vi "Teleop.vi"(10 "Match Info":T5={"Autonomous Elapsed Seconds"=0.0, "TeleOp Elapsed Seconds"=0.0, "Disabled Elapsed Seconds"=0.0, "Visited Autonomous"=FALSE, "Visited TeleOp"=FALSE, "Visited Disabled"=FALSE, "Autonomous Settings"={"Autonomous Style"=enum."Independent", "VI Refnum"=refnum}}, 11 "Call Context":T6) -> ()   [LabVIEW 2013]
doc: "This VI is called for each TeleOp packet received from the DS where the robot is not disabled. It is often used to read from the joysticks and update I/O or to update setpoints for timed control loops. It should complete and return within 20 milliseconds or it may miss DS packets."
uses:
  <vilib>/Rock Robotics/WPI/DriverStation/WPI_DriverStationDerivedRobotMode.ctl
  <vilib>/Rock Robotics/WPI/DriverStation/WPI_DriverStationMatch Info.ctl
  <vilib>/Rock Robotics/WPI/Joystick/WPI_JoystickButtonState.ctl
  <vilib>/Rock Robotics/WPI/Solenoid/WPI_SolenoidValue.ctl
  <vilib>/Rock Robotics/WPI/Relay/WPI_RelayValue.ctl
  Robot Global Data.vi
  <vilib>/Rock Robotics/Network Tables/SD Read Number.vi
  <vilib>/Rock Robotics/WPI/Solenoid/WPI_SolenoidGetEnum.vi
  <vilib>/Rock Robotics/WPI/Solenoid/Deprecated/WPI_SolenoidGetBool.vi
  <vilib>/Rock Robotics/WPI/Compressor/WPI_CompressorGetSetRefNum.vi
  <vilib>/Rock Robotics/WPI/Solenoid/WPI_SolenoidSetEnum.vi
  <vilib>/Rock Robotics/WPI/Joystick/WPI_JoystickGetSetRefNum.vi
  <vilib>/Rock Robotics/WPI/RobotDrive/WPI_RobotDriveGetSetRefNum.vi
panel:
  out "Waveform Chart 3":dbl(graph)
  out "Buttons":T1
  out "Axes":T2
  out "Firing Pin on off":bool
  out "Reed Switch 2":bool
  out "Reed Switch 1":bool
  out "Top Limit Tripped":bool
  out "Micro Switch":bool
  out "Bottom Limit Tripped":bool
  in  "Grabber Axis Value":T3(ring)
  out "Waveform Chart 2":dbl(graph)
  in  "OK Button":bool
  in  "Set Point":dbl
  in  "Run Grabber PID":bool
  in  "Current Shooter Status":T4(ring)
  out "Waveform Chart":dbl(graph)
  out "Mechanism Moving Up":bool
  out "Mechanism Moving Down":bool
  out "Time Since Button Pressed":dbl
  in  "Manual Override Activated":bool
  in  "Button 8 Pressed":bool
  in  "Button 3 Pressed":bool
  in  "Button 2 Pressed":bool
  in  "Tick Taken":bool
  out "Time at Gather":dbl
  out "Timer for firing mech":dbl
  in  "Mechanism Status":string
  # "Joystick Debug"
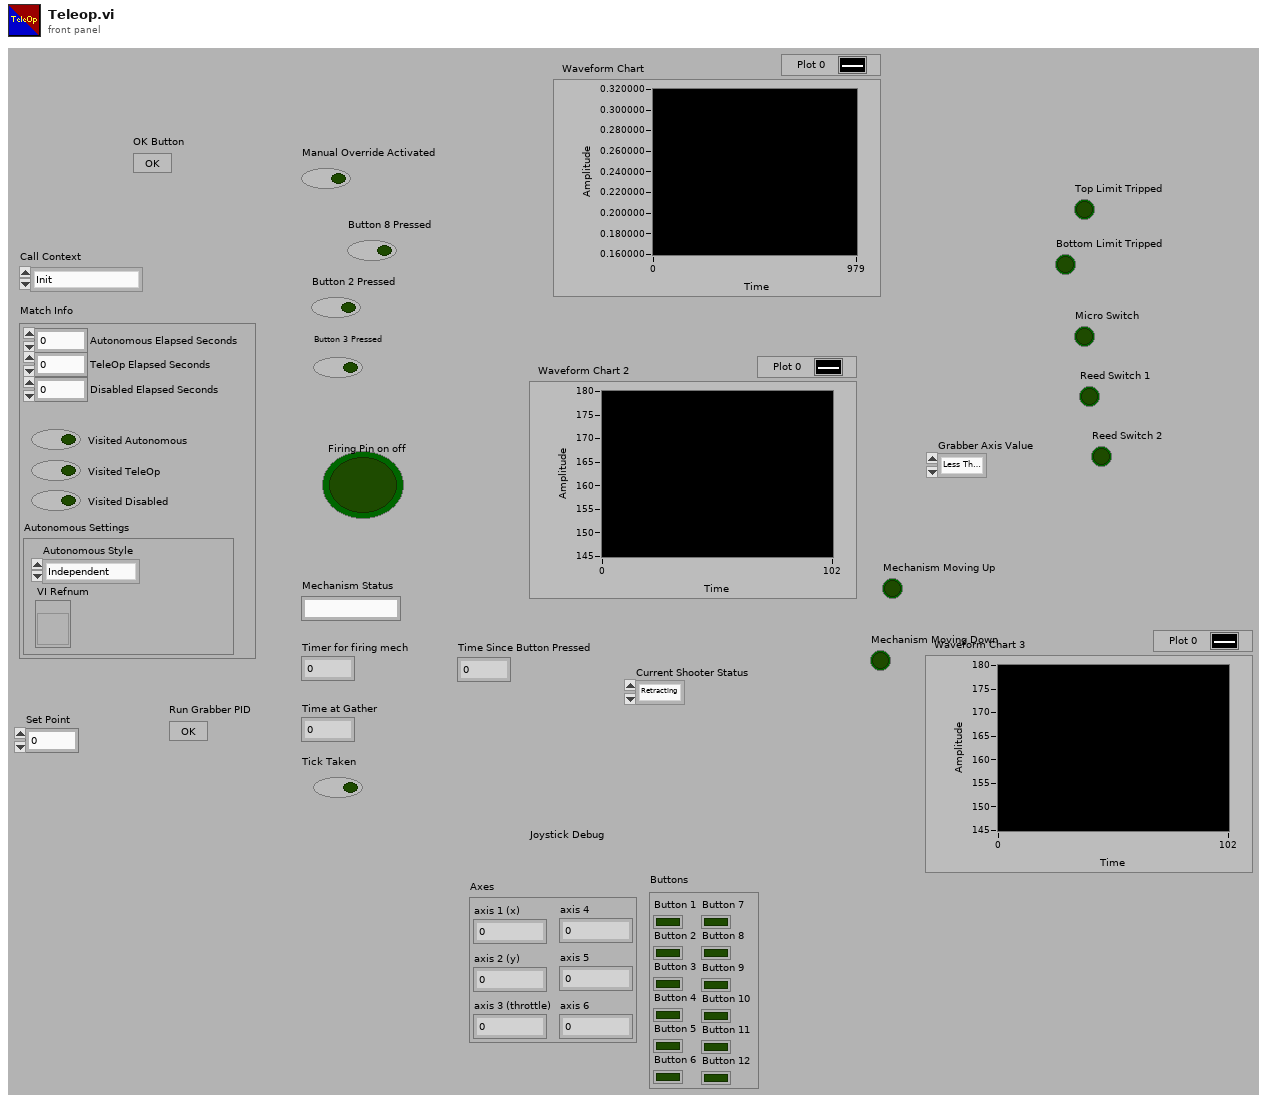
[diagram p1: front panel]
types:
  T1 = typedef "WPI_JoystickButtonState.ctl" = cluster{"Button 1":bool, "Button 2":bool, "Button 3":bool, "Button 4":bool, "Button 5":bool, "Button 6":bool, "Button 7":bool, "Button 8":bool, "Button 9":bool, "Button 10":bool, "Button 11":bool, "Button 12":bool}
  T2 = cluster{"axis 1 (x)":dbl, "axis 2 (y)":dbl, "axis 3 (throttle)":dbl, "axis 4":dbl, "axis 5":dbl, "axis 6":dbl}
  T3 = enum16{"Less Than Zero", "Greater Than Zero", "Equal To Zero"}
  T4 = enum16{"Retracting", "Firing", "Ready to fire", "Pulling back", "Just fired"}
  T5 = typedef "WPI_DriverStationMatch Info.ctl" = cluster{"Autonomous Elapsed Seconds":dbl, "TeleOp Elapsed Seconds":dbl, "Disabled Elapsed Seconds":dbl, "Visited Autonomous":bool, "Visited TeleOp":bool, "Visited Disabled":bool, "Autonomous Settings":cluster{"Autonomous Style":enum16{"Iterative", "Independent"}, "VI Refnum":refnum<vi>}}
  T6 = typedef "WPI_DriverStationDerivedRobotMode.ctl" = enum16{"Init", "Execute", "Stop"}
  T7 = typedef "WPI_SolenoidValue.ctl" = enum16{"Off", "On", "Forward", "Reverse"}
  T8 = typedef "WPI_MotorControlDeviceRef.ctl" = cluster{"DeviceStatus":errorcluster, "Type":enum16{"PWM", "CAN"}, "PWM":cluster{"Digital Module":T9, "PWM Channel":T10, "DeadBand":T11}, "CAN":cluster{"Device Number":u8, "Control Mode":T12, "Semaphore":T13, "Max Vout":dbl}, "Invert":bool, "TransformRef":T14, "InvTransformRef":T14}
  T9 = typedef "FPGA_TypedefDigitalModule.ctl" = enum16{"Digital Module 1", "Digital Module 2"}
  T10 = typedef "FPGA_DIOPWMChannel.ctl" = enum8{"PWM 1", "PWM 2", "PWM 3", "PWM 4", "PWM 5", "PWM 6", "PWM 7", "PWM 8", "PWM 9", "PWM 10", "Invalid"}
  T11 = typedef "WPI_PWMDeadband.ctl" = cluster{"Name":string, "maxPositivePwm":i32, "minPositivePwm":i32, "centerPwm":i32, "maxNegativePwm":i32, "minNegativePwm":i32, "angularRange":u16}
  T12 = typedef "WPI_CANJaguar_ControlMode.ctl" = enum8{"Percent VBus", "Current", "Speed", "Position", "Voltage"}
  T13 = typedef "Semaphore RefNum" = refnum<k1>
  T14 = typedef "WPI_PWMTransform_ConPane.ctl" = refnum<vi>
  T15 = typedef "WPI_EncoderDevRef.ctl" = cluster{"DevStatus":errorcluster, "EncoderIndex":T16, "CounterIndex":T17, "DistancePerCount":dbl, "Decoding Type":T18}
  T16 = typedef "FPGA_EncoderIdx.ctl" = enum8{"Enc 0", "Enc 1", "Enc 2", "Enc 3", "Invalid"}
  T17 = typedef "FPGA_CounterCtrSystemIndex.ctl" = enum8{"Ctr 0", "Ctr 1", "Ctr 2", "Ctr 3", "Ctr 4", "Ctr 5", "Ctr 6", "Ctr 7", "Invalid"}
  T18 = typedef "WPI_EncoderType.ctl" = enum16{"1x", "2x", "4x"}
  T19 = typedef "WPI_JoystickDevRef.ctl" = cluster{"Device":T20}
  T20 = typedef "WPI_JoystickDeviceEnum.ctl" = enum16{"USB 1", "USB 2", "USB 3", "USB 4", "Kinect 1", "Kinect 2"}
  T21 = typedef "WPI_SolenoidDevRef.ctl" = cluster{"DevStatus":errorcluster, "Solenoid Module":T22, "Forward Solenoid Channel":T23, "Reverse Solenoid Channel":T23}
  T22 = typedef "FPGA_TypedefSolenoidModule.ctl" = enum16{"Solenoid Module 1", "Solenoid Module 2"}
  T23 = typedef "WPI_SolenoidChannel.ctl" = enum8{"Solenoid 1", "Solenoid 2", "Solenoid 3", "Solenoid 4", "Solenoid 5", "Solenoid 6", "Solenoid 7", "Solenoid 8", "Invalid"}
  T24 = typedef "WPI_RelayDevRef.ctl" = cluster{"DevStatus":errorcluster, "Relay Channel":T25, "Digital Module":T9, "Relay Direction":T26}
  T25 = typedef "FPGA_DIORelayChannel.ctl" = enum8{"Relay 1", "Relay 2", "Relay 3", "Relay 4", "Relay 5", "Relay 6", "Relay 7", "Relay 8", "Invalid"}
  T26 = typedef "WPI_RelayDirection.ctl" = enum16{"Both directions", "Forward only", "Reverse only"}
  T27 = typedef "WPI_DigitalInputDevRef.ctl" = cluster{"DevStatus":errorcluster, "DIO Channel":T28, "Digital Module":T9}
  T28 = typedef "FPGA_DIOChannel.ctl" = enum8{"DIO 1", "DIO 2", "DIO 3", "DIO 4", "DIO 5", "DIO 6", "DIO 7", "DIO 8", "DIO 9", "DIO 10", "DIO 11", "DIO 12", "DIO 13", "DIO 14", "Invalid"}
  T29 = typedef "WPI_CompressorDevRef.ctl" = cluster{"DevStatus":errorcluster, "DigitalInputDevRef":T27, "RelayDevRef":T24}
  T30 = typedef "WPI_RelayValue.ctl" = enum16{"Off", "On", "Forward", "Reverse"}
  T31 = typedef "WPI_AnalogChannelDevRef.ctl" = cluster{"DevStatus":errorcluster, "Analog Module":T32, "Analog Channel":T33}
  T32 = typedef "FPGA_TypedefAnalogModule.ctl" = enum16{"Analog Module 1", "Analog Module 2"}
  T33 = typedef "FPGA_AIChannel.ctl" = enum8{"AI 1", "AI 2", "AI 3", "AI 4", "AI 5", "AI 6", "AI 7", "AI 8", "Invalid"}
  T34 = typedef "WPI_ServoDeviceRef.ctl" = cluster{"DeviceStatus":errorcluster, "Digital Module":T9, "PWM Channel":T10, "DeadBand":T11}
  T35 = typedef "WPI_RobotDriveDevRef.ctl" = cluster{"DevStatus":errorcluster, "Motors[]":T8[], "Square Inputs":bool, "Max Output":dbl, "Isochronous":bool}
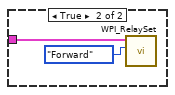
[diagram p8: hidden frame]
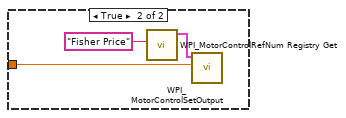
[diagram p9: hidden frame]
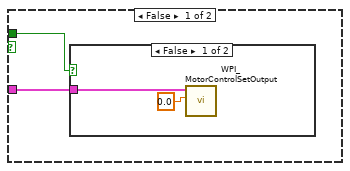
[diagram p10: hidden frame]
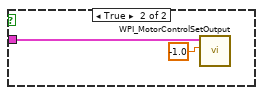
[diagram p11: hidden frame]
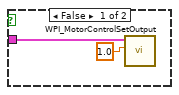
[diagram p12: hidden frame]
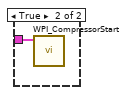
[diagram p13: hidden frame]
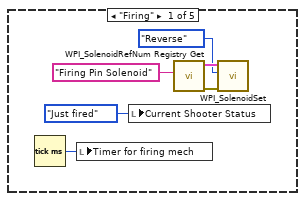
[diagram p16: hidden frame]
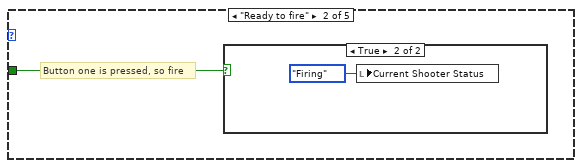
[diagram p17: hidden frame]
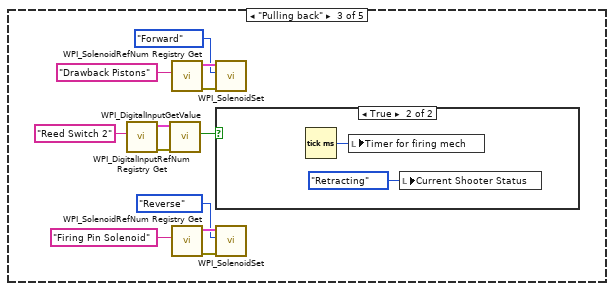
[diagram p19: hidden frame]
diagram:
  (unwired) "This code sets the toggle rate used by the Periodic Tasks VI.  For teleop mode we flash the USER1 LED on the cRIO at a fast rate.  Look at the Periodic Tasks VI to see how this global value is used."
  (unwired) "This VI is called each time a TeleOp DS packet is received.  Use it to respond to new joystick or Driver Station values.\n\nCommon tasks include reading the joysticks and updating motors, and updating setpoints for periodic loops.\n\nYou can open I/O on the FIRST Call, or in the Begin.vi."
  # "TOP LIMIT SWITCH IS INVERTED"
  # "Check me!"
  # "These are examples of reading dashboard variables."
  # "Publish the Robot Drive Motor\nvalues to the dashboard"
  # "Publish the joystick data the\nrobot sees to the dashboard"
  # "Each time we enter, report that\nwe are running teleop"
  # "Use to differentiate between\nFirst, Last, and Intermediate calls"
  # "This can help determine what has\nbeen run and for how long"
  # "Read Joystick X and Y values and update motor values"
  n1 = disable-structure shown="Disabled" {
    frame Disabled {
      n2 = case shown="True" {
        selector: _ -> [_ _]
        frame False {
        }
        frame True {
          n3 = local read "Run Grabber PID"() -> (w130:bool)
          n4 = case shown="True" w130 {
            frame False {
            }
            frame True {
              # "one encoder"
              n5 = call "grabberpidinit.vi"("setpoint"="Set Point") -> ("Done? 2"=w136:bool, "output"=w135:dbl)  [unwired: 9 in]
              n6 = Not(x=w136) -> (.not. x?=w140:bool)
              n7 = call <vilib>:"WPI_MotorControlRefNum Registry Get.vi"("refnum name"="Fisher Price") -> ("MotorControlDevRef"=w137:T8)  [unwired: 9 in, 1 out]
              n8 = case shown="True" w136 {
                frame False {
                }
                frame True {
                  n9 = call <vilib>:"WPI_EncoderRefNum Registry Get.vi"("refnum name"="Tough Box Encoder") -> ("EncoderDevRef"=w141:T15)  [unwired: 9 in, 1 out]
                  n10 = call <vilib>:"WPI_EncoderReset.vi"("EncoderDevRef"=w141) -> ()  [unwired: 9 in, 2 out]
                }
              }
              n11 = call <vilib>:"WPI_EncoderRefNum Registry Get.vi"("refnum name"="Tough Box Encoder") -> ("error out"=w134:errorcluster, "EncoderDevRef"=w133:T15)  [unwired: 9 in]
              n12 = call <vilib>:"WPI_MotorControlSetOutput.vi"("Output"=w135, "MotorControlDevRef"=w137) -> ()  [unwired: 7 in, 3 out]
              n13 = local write "Run Grabber PID"(w140) -> ()
              n14 = call <vilib>:"WPI_EncoderGet.vi"("error in (no error)"=w134, "EncoderDevRef"=w133) -> ("Distance"=w131:dbl)  [unwired: 4 in, 5 out]
            }
          }
        }
      }
    }
    frame Enabled {
    }
  }
  n15 = disable-structure shown="Disabled" {
    frame Disabled {
      n16 = call <vilib>:"WPI_JoystickRefNum Registry Get.vi"("refnum name"="Joystick 1") -> ("JoystickDevRef"=w145:T19)  [unwired: 1 in, 9 out]
      n17 = call <vilib>:"WPI_JoystickGet.vi"("JoystickDevRef"=w145) -> ("Buttons"=w144:T1)  [unwired: 1 in, 5 out]
      n18 = Unbundle By Name(w144) -> ("Button 4"=w143:bool)
      n19 = case shown="True" w143 {
        frame False {
        }
        frame True {
          n20 = call <vilib>:"WPI_MotorControlRefNum Registry Get.vi"("refnum name"="Snowblower") -> ("MotorControlDevRef"=w150:T8)  [unwired: 9 in, 1 out]
          n21 = call <vilib>:"WPI_MotorControlSetOutput.vi"("Output"=-7.0, "MotorControlDevRef"=w150) -> ()  [unwired: 7 in, 3 out]
          n22 = call <vilib>:"WPI_SolenoidRefNum Registry Get.vi"("refnum name"="Grabber Pistons Solenoid") -> ("SolenoidDevRef"=w147:T21)  [unwired: 9 in, 1 out]
          n23 = call-poly <vilib>:"WPI_SolenoidSet.vi"("Value"=WPI_SolenoidValue."Reverse", "SolenoidDevRef"=w147) -> ()  [unwired: 8 in, 2 out]
        }
      }
    }
    frame Enabled {
    }
  }
  n24 = call <vilib>:"WPI_DriverStationReport Robot Code State.vi"("TeleOp"=TRUE ("Autonomous")) -> ()  [unwired: 10 in, 1 out]
  n25 = global write "Robot Global Data.vi" "LED toggle rate (ms)"(u32 100 ("LED ms toggle rate")) -> ()
  n26 = case shown="True" "OK Button" {
    frame False {
    }
    frame True {
      n27 = local write "Run Grabber PID"(TRUE) -> ()
    }
  }
  n28 = Unbundle By Name("Match Info") -> ()  [unwired: 1 out]
  n29 = call <vilib>:"SD Read Boolean.vi"("Name"="Light Ring On") -> ("Boolean"=w37:bool)  [unwired: 8 in, 2 out]
  n30 = call <vilib>:"WPI_RelayRefNum Registry Get.vi"("refnum name"="Light Ring") -> ("RelayDevRef"=w36:T24)  [unwired: 9 in, 1 out]
  n31 = call <vilib>:"WPI_DigitalInputRefNum Registry Get.vi"("refnum name"="Reed Switch 1") -> ("DigitalInputDevRef"=w56:T27)  [unwired: 9 in, 1 out]
  n32 = call <vilib>:"WPI_DigitalInputRefNum Registry Get.vi"("refnum name"="Reed Switch 2") -> ("DigitalInputDevRef"=w49:T27)  [unwired: 9 in, 1 out]
  n33 = call <vilib>:"WPI_DigitalInputRefNum Registry Get.vi"("refnum name"="Reed Switch 2") -> ("DigitalInputDevRef"=w53:T27)  [unwired: 9 in, 1 out]
  n34 = call <vilib>:"WPI_DigitalInputRefNum Registry Get.vi"("refnum name"="Micro Switch 1") -> ("DigitalInputDevRef"=w69:T27)  [unwired: 9 in, 1 out]
  n35 = call <vilib>:"WPI_DigitalInputRefNum Registry Get.vi"("refnum name"="Micro Switch 1") -> ("DigitalInputDevRef"=w45:T27)  [unwired: 9 in, 1 out]
  n36 = call <vilib>:"WPI_DigitalInputRefNum Registry Get.vi"("refnum name"="Top Limit Switch") -> ("DigitalInputDevRef"=w62:T27)  [unwired: 9 in, 1 out]
  n37 = call <vilib>:"WPI_SolenoidRefNum Registry Get.vi"("refnum name"="Firing Pin Solenoid") -> ("SolenoidDevRef"=w29:T21)  [unwired: 9 in, 1 out]
  n38 = call <vilib>:"SD Read Boolean.vi"("Name"="Compressor On/Off") -> ("Boolean"=w71:bool)  [unwired: 8 in, 2 out]
  n39 = call <vilib>:"WPI_CompressorRefNum Registry Get.vi"("refnum name"="Compressor") -> ("CompressorDevRef"=w72:T29)  [unwired: 9 in, 1 out]
  n40 = call <vilib>:"WPI_DigitalInputRefNum Registry Get.vi"("refnum name"="Bottom Limit Switch") -> ("DigitalInputDevRef"=w77:T27)  [unwired: 9 in, 1 out]
  n41 = case shown="False" w37 {
    tunnel: w36 -> [w154 w157]
    frame False {
      n42 = call <vilib>:"WPI_RelaySet.vi"("RelayValue"=WPI_RelayValue."Off", "RelayDevRef"=w154) -> ()  [unwired: 8 in, 2 out]
    }
    frame True {
      n43 = call <vilib>:"WPI_RelaySet.vi"("RelayValue"=WPI_RelayValue."Forward", "RelayDevRef"=w157) -> ()  [unwired: 8 in, 2 out]
    }
  }
  n44 = call <vilib>:"WPI_DigitalInputGetValue.vi"("DigitalInputDevRef"=w56) -> ("Value"=→"Reed Switch 1":bool)  [unwired: 8 in, 2 out]
  n45 = call <vilib>:"WPI_DigitalInputGetValue.vi"("DigitalInputDevRef"=w49) -> ("Value"=w48:bool)  [unwired: 8 in, 2 out]
  n46 = call <vilib>:"WPI_DigitalInputGetValue.vi"("DigitalInputDevRef"=w53) -> ("Value"=→"Reed Switch 2":bool)  [unwired: 8 in, 2 out]
  n47 = call <vilib>:"WPI_DigitalInputGetValue.vi"("DigitalInputDevRef"=w69) -> ("Value"=→"Micro Switch":bool)  [unwired: 8 in, 2 out]
  n48 = call <vilib>:"WPI_DigitalInputGetValue.vi"("DigitalInputDevRef"=w45) -> ("Value"=w44:bool)  [unwired: 8 in, 2 out]
  n49 = call <vilib>:"WPI_DigitalInputGetValue.vi"("DigitalInputDevRef"=w62) -> ("Value"=→"Top Limit Tripped":bool)  [unwired: 8 in, 2 out]
  n50 = call <vilib>:"WPI_AnalogChannelRefNum Registry Get.vi"("refnum name"="Grabber Ultrasonic Sensor") -> ("AIDeviceRef"=w34:T31)  [unwired: 9 in, 1 out]
  n51 = case shown="False" w71 {
    tunnel: w72 -> [w158 w159]
    frame False {
      n52 = call <vilib>:"WPI_CompressorStop.vi"("CompressorDevRef"=w158) -> ()  [unwired: 9 in, 2 out]
    }
    frame True {
      n53 = call <vilib>:"WPI_CompressorStart.vi"("CompressorDevRef"=w159) -> ()  [unwired: 9 in, 2 out]
    }
  }
  n54 = call <vilib>:"WPI_DigitalInputGetValue.vi"("DigitalInputDevRef"=w77) -> ("Value"=→"Bottom Limit Tripped":bool)  [unwired: 8 in, 2 out]
  n55 = Not(x=w48) -> (.not. x?=w47:bool)
  n56 = call-poly <vilib>:"SD Read Value.vi"("Name"="Camera Pitch Control") -> ("Numeric"=w91:dbl)  [unwired: 8 in, 2 out]
  n57 = call <vilib>:"WPI_SolenoidRefNum Registry Get.vi"("refnum name"="Firing Pin Solenoid") -> ("SolenoidDevRef"=w102:T21)  [unwired: 9 in, 1 out]
  n58 = call <vilib>:"SD Read Boolean.vi"("Name"="Manual Mechanism Override") -> ("Boolean"=w57:bool)  [unwired: 8 in, 2 out]
  n59 = call <vilib>:"WPI_SolenoidRefNum Registry Get.vi"("refnum name"="Drawback Pistons") -> ("SolenoidDevRef"=w100:T21)  [unwired: 9 in, 1 out]
  n60 = call <vilib>:"WPI_SolenoidRefNum Registry Get.vi"("refnum name"="Grabber Pistons Solenoid") -> ("SolenoidDevRef"=w78:T21)  [unwired: 9 in, 1 out]
  n61 = call-poly <vilib>:"WPI_SolenoidGet.vi"("SolenoidDevRef"=w29) -> ("Value"=→"Firing Pin on off":bool)  [unwired: 8 in, 2 out]
  n62 = Not(x=w44) -> (.not. x?=w43:bool)
  n63 = call <vilib>:"WPI_ServoRefNum Registry Get.vi"("refnum name"="Camera Pitch Servo") -> ("ServoDeviceRef"=w92:T34)  [unwired: 9 in, 1 out]
  n64 = call-poly <vilib>:"SD Read Value.vi"("Name"="Camera Rotation Control") -> ("Numeric"=w95:dbl)  [unwired: 8 in, 2 out]
  n65 = call <vilib>:"WPI_AnalogChannelGetVoltage.vi"("AIDeviceRef"=w34) -> ("Voltage"=→"Waveform Chart":dbl)  [unwired: 8 in, 2 out]
  n66 = call <vilib>:"WPI_ServoRefNum Registry Get.vi"("refnum name"="Camera Rotation Servo") -> ("ServoDeviceRef"=w94:T34)  [unwired: 9 in, 1 out]
  n67 = call <vilib>:"SD Write Boolean.vi"("Boolean"=w47, "Name"="Are Drawback Pistons Extended") -> ()  [unwired: 8 in, 2 out]
  n68 = call <vilib>:"SD Write Boolean.vi"("Boolean"=w43, "Name"="Is The Firing Pin Piston Extended") -> ()  [unwired: 8 in, 2 out]
  n69 = call <vilib>:"SD Read Boolean.vi"("Name"="Manual Mechanism Override") -> ("Boolean"=w85:bool)  [unwired: 8 in, 2 out]
  n70 = case shown="True" w57 {
    tunnel: w102 -> [_ w178]
    tunnel: w100 -> [_ w177]
    tunnel: w78 -> [_ w160]
    frame False {
    }
    frame True {
      n71 = call <vilib>:"SD Read Boolean.vi"("Name"="Firing Pin Piston Extended") -> ("Boolean"=w175:bool)  [unwired: 8 in, 2 out]
      n72 = call <vilib>:"SD Read Boolean.vi"("Name"="Drawback Pistons Activated") -> ("Boolean"=w161:bool)  [unwired: 8 in, 2 out]
      n73 = call <vilib>:"SD Read Boolean.vi"("Name"="Grabber Pistons Extended") -> ("Boolean"=w169:bool)  [unwired: 8 in, 2 out]
      n74 = case shown="True" w161 {
        tunnel: w177 -> [_ w186]
        frame False {
        }
        frame True {
          n75 = call <vilib>:"SD Read Boolean.vi"("Name"="Drawback Piston Extended") -> ("Boolean"=w184:bool)  [unwired: 8 in, 2 out]
          n76 = Equal?(x=w184, y=FALSE) -> (x = y?=w182:bool)
          n77 = Select(t=WPI_SolenoidValue."Forward" ("Value"), s=w182, f=WPI_SolenoidValue."Reverse") -> (s? t:f=w179:T7)
          n78 = call-poly <vilib>:"WPI_SolenoidSet.vi"("Value"=w179, "SolenoidDevRef"=w186) -> ()  [unwired: 8 in, 2 out]
        }
      }
      n79 = Equal?(x=w175, y=FALSE) -> (x = y?=w171:bool)
      n80 = Equal?(x=w169, y=FALSE) -> (x = y?=w167:bool)
      n81 = Select(t=WPI_SolenoidValue."Forward" ("Value"), s=w171, f=WPI_SolenoidValue."Reverse") -> (s? t:f=w172:T7)
      n82 = Select(t=WPI_SolenoidValue."Forward" ("Value"), s=w167, f=WPI_SolenoidValue."Reverse") -> (s? t:f=w164:T7)
      n83 = call-poly <vilib>:"WPI_SolenoidSet.vi"("Value"=w172, "SolenoidDevRef"=w178) -> ()  [unwired: 8 in, 2 out]
      n84 = call-poly <vilib>:"WPI_SolenoidSet.vi"("Value"=w164, "SolenoidDevRef"=w160) -> ()  [unwired: 8 in, 2 out]
    }
  }
  n85 = call-poly <vilib>:"WPI_SolenoidGet.vi"("SolenoidDevRef"=w78) -> ("Value"=w80:T7)  [unwired: 8 in, 2 out]
  n86 = call <vilib>:"WPI_JoystickRefNum Registry Get.vi"("refnum name"="Joystick 1") -> ("JoystickDevRef"=w110:T19)  [unwired: 1 in, 9 out]
  n87 = call <vilib>:"WPI_JoystickRefNum Registry Get.vi"("refnum name"="Joystick 1") -> ("JoystickDevRef"=w113:T19)  [unwired: 1 in, 9 out]
  n88 = call <vilib>:"WPI_ServoSetAngle.vi"("Angle"=w91, "ServoDeviceRef"=w92) -> ()  [unwired: 8 in, 2 out]
  n89 = call <vilib>:"WPI_ServoSetAngle.vi"("Angle"=w95, "ServoDeviceRef"=w94) -> ()  [unwired: 8 in, 2 out]
  n90 = Equal?(x=w80, y=WPI_SolenoidValue."Forward") -> (x = y?=w32:bool)
  n91 = call <vilib>:"WPI_JoystickGet.vi"("JoystickDevRef"=w110) -> ("Buttons"=w109:T1)  [unwired: 1 in, 5 out]
  n92 = Not(x=w32) -> (.not. x?=w31:bool)
  n93 = Unbundle By Name(w109) -> ("Button 8"=w108:bool)
  n94 = call <vilib>:"SD Read Boolean.vi"("Name"="Drawback Pistons Activated") -> ("Boolean"=w66:bool)  [unwired: 8 in, 2 out]
  n95 = Not(x=w85) -> (.not. x?=w65:bool)
  n96 = call <vilib>:"SD Write Boolean.vi"("Boolean"=w31, "Name"="Are Grabber Pistons Extended") -> ()  [unwired: 8 in, 2 out]
  n97 = call <vilib>:"WPI_JoystickGet.vi"("JoystickDevRef"=w113) -> ("Buttons"=w112:T1, "Axes"=w107:T2)  [unwired: 1 in, 4 out]
  n98 = case shown="True" w108 {
    frame False {
    }
    frame True {
      n99 = global read "Robot Global Data.vi" "Time since  button 8 pressed"() -> (w187:dbl)
      n100 = Tick Count (ms)() -> (millisecond timer value=w191:u32)
      n101 = Subtract(x=w191, y=w187) -> (x-y=w190:dbl)
      n102 = Greater?(x=w190, y=300) -> (0:w188:bool)
      n103 = case shown="True" w188 {
        frame False {
        }
        frame True {
          n104 = Tick Count (ms)() -> (millisecond timer value=w194:u32)
          n105 = local read "Manual Override Activated"() -> (w192:bool)
          n106 = global write "Robot Global Data.vi" "Time since  button 8 pressed"(w194) -> ()
          n107 = Not(x=w192) -> (.not. x?=w193:bool)
          n108 = local write "Manual Override Activated"(w193) -> ()
        }
      }
    }
  }
  n109 = Unbundle By Name(w107) -> ("axis 4"=w60:dbl)
  n110 = call <vilib>:"WPI_JoystickRefNum Registry Get.vi"("refnum name"="Joystick 1") -> ("JoystickDevRef"=w125:T19)  [unwired: 1 in, 9 out]
  n111 = Unbundle By Name(w112) -> ("Button 1"=w84:bool, "Button 5"=w41:bool, "Button 6"=w42:bool)  [unwired: 2 out]
  n112 = And(x=w65, y=w66) -> (x .and. y?=w64:bool)
  n113 = call <vilib>:"WPI_DigitalInputRefNum Registry Get.vi"("refnum name"="Micro Switch 1") -> ("DigitalInputDevRef"=w21:T27)  [unwired: 9 in, 1 out]
  n114 = call <vilib>:"WPI_MotorControlRefNum Registry Get.vi"("refnum name"="Snowblower") -> ("MotorControlDevRef"=w40:T8)  [unwired: 9 in, 1 out]
  n115 = call <vilib>:"WPI_JoystickGet.vi"("JoystickDevRef"=w125) -> ("Buttons"=w123:T1, "Axes"=w120:T2)  [unwired: 1 in, 4 out]
  "Axes" <- w120
  "Buttons" <- w123
  n116 = Unbundle By Name(w120) -> ("axis 1 (x)"=w90:dbl, "axis 2 (y)"=w88:dbl)  [unwired: 1 out]
  n117 = Cluster To Array(cluster=w123) -> (array=w122:bool[])
  n118 = Cluster To Array(cluster=w120) -> (array=w119:dbl[])
  n119 = case shown="True" w64 {
    tunnel: w84 -> [_ w195]
    frame False {
    }
    frame True {
      n120 = case shown="\"Retracting\"" "Current Shooter Status" {
        tunnel: w195 -> [_ w203 _ _ _]
        frame "Firing" {
          n121 = Tick Count (ms)() -> (millisecond timer value=w197:u32)
          n122 = local write "Timer for firing mech"(w197) -> ()
          n123 = local write "Current Shooter Status"(T4."Just fired" ("Current Shooter Status")) -> ()
          n124 = call <vilib>:"WPI_SolenoidRefNum Registry Get.vi"("refnum name"="Firing Pin Solenoid") -> ("error out"=w201:errorcluster, "SolenoidDevRef"=w200:T21)  [unwired: 9 in]
          n125 = call-poly <vilib>:"WPI_SolenoidSet.vi"("error in (no error)"=w201, "Value"=WPI_SolenoidValue."Reverse", "SolenoidDevRef"=w200) -> ()  [unwired: 7 in, 2 out]
        }
        frame "Ready to fire" {
          # "Button one is pressed, so fire"
          n126 = case shown="True" w203 {
            frame False {
            }
            frame True {
              n127 = local write "Current Shooter Status"(T4."Firing" ("Current Shooter Status")) -> ()
            }
          }
        }
        frame "Pulling back" {
          n128 = call <vilib>:"WPI_DigitalInputRefNum Registry Get.vi"("refnum name"="Reed Switch 2") -> ("error out"=w206:errorcluster, "DigitalInputDevRef"=w207:T27)  [unwired: 9 in]
          n129 = call <vilib>:"WPI_DigitalInputGetValue.vi"("error in (no error)"=w206, "DigitalInputDevRef"=w207) -> ("Value"=w205:bool)  [unwired: 7 in, 2 out]
          n130 = call <vilib>:"WPI_SolenoidRefNum Registry Get.vi"("refnum name"="Drawback Pistons") -> ("error out"=w211:errorcluster, "SolenoidDevRef"=w210:T21)  [unwired: 9 in]
          n131 = call <vilib>:"WPI_SolenoidRefNum Registry Get.vi"("refnum name"="Firing Pin Solenoid") -> ("error out"=w215:errorcluster, "SolenoidDevRef"=w214:T21)  [unwired: 9 in]
          n132 = call-poly <vilib>:"WPI_SolenoidSet.vi"("error in (no error)"=w211, "Value"=WPI_SolenoidValue."Forward", "SolenoidDevRef"=w210) -> ()  [unwired: 7 in, 2 out]
          n133 = case shown="True" w205 {
            frame False {
            }
            frame True {
              n134 = Tick Count (ms)() -> (millisecond timer value=w217:u32)
              n135 = local write "Timer for firing mech"(w217) -> ()
              n136 = local write "Current Shooter Status"(T4."Retracting" ("Current Shooter Status")) -> ()
            }
          }
          n137 = call-poly <vilib>:"WPI_SolenoidSet.vi"("error in (no error)"=w215, "Value"=WPI_SolenoidValue."Reverse", "SolenoidDevRef"=w214) -> ()  [unwired: 7 in, 2 out]
        }
        frame "Retracting" {
          n138 = local read "Timer for firing mech"() -> (w232:dbl)
          n139 = call <vilib>:"WPI_DigitalInputRefNum Registry Get.vi"("refnum name"="Reed Switch 1") -> ("error out"=w224:errorcluster, "DigitalInputDevRef"=w225:T27)  [unwired: 9 in]
          n140 = call <vilib>:"WPI_DigitalInputGetValue.vi"("error in (no error)"=w224, "DigitalInputDevRef"=w225) -> ("Value"=w220:bool)  [unwired: 7 in, 2 out]
          n141 = call <vilib>:"WPI_SolenoidRefNum Registry Get.vi"("refnum name"="Firing Pin Solenoid") -> ("error out"=w235:errorcluster, "SolenoidDevRef"=w234:T21)  [unwired: 9 in]
          n142 = call-poly <vilib>:"WPI_SolenoidSet.vi"("error in (no error)"=w235, "Value"=WPI_SolenoidValue."Forward", "SolenoidDevRef"=w234) -> ()  [unwired: 7 in, 2 out]
          n143 = Not(x=w220) -> (.not. x?=w219:bool)
          n144 = Tick Count (ms)() -> (millisecond timer value=w229:u32)
          n145 = case shown="True" w219 {
            frame False {
            }
            frame True {
              n146 = local write "Current Shooter Status"(T4."Ready to fire" ("Current Shooter Status")) -> ()
            }
          }
          n147 = Subtract(x=w229, y=w232) -> (x-y=w231:dbl)
          n148 = Greater Or Equal?(x=1000, y=w231) -> (x >= y?=w222:bool)
          n149 = call <vilib>:"WPI_SolenoidRefNum Registry Get.vi"("refnum name"="Drawback Pistons") -> ("SolenoidDevRef"=w227:T21)  [unwired: 9 in, 1 out]
          n150 = And(x=TRUE, y=w222) -> (x .and. y?=w223:bool)
          n151 = case shown="True" w223 {
            tunnel: w227 -> [_ w238]
            frame False {
            }
            frame True {
              n152 = call-poly <vilib>:"WPI_SolenoidSet.vi"("Value"=WPI_SolenoidValue."Reverse", "SolenoidDevRef"=w238) -> ()  [unwired: 8 in, 2 out]
            }
          }
        }
        frame "Just fired", Default {
          # "When MicroSwitch is \nadded, Change this \nto read from that"
          n153 = local read "Timer for firing mech"() -> (w250:dbl)
          n154 = call <vilib>:"WPI_SolenoidRefNum Registry Get.vi"("refnum name"="Firing Pin Solenoid") -> ("error out"=w245:errorcluster, "SolenoidDevRef"=w244:T21)  [unwired: 9 in]
          n155 = Tick Count (ms)() -> (millisecond timer value=w247:u32)
          n156 = call-poly <vilib>:"WPI_SolenoidSet.vi"("error in (no error)"=w245, "Value"=WPI_SolenoidValue."Reverse", "SolenoidDevRef"=w244) -> ()  [unwired: 7 in, 2 out]
          n157 = Subtract(x=w247, y=w250) -> (x-y=w249:dbl)
          n158 = Greater Or Equal?(x=3000, y=w249) -> (x >= y?=w242:bool)
          n159 = And(x=TRUE, y=w242) -> (x .and. y?=w241:bool)
          n160 = case shown="True" w241 {
            frame False {
            }
            frame True {
              n161 = local write "Current Shooter Status"(T4."Pulling back" ("Current Shooter Status")) -> ()
            }
          }
        }
      }
    }
  }
  n162 = case shown="True" w42 {
    tunnel: w41 -> [w253 w259]
    tunnel: w40 -> [w252 w258]
    frame False {
      n163 = case shown="False" w253 {
        tunnel: w252 -> [w255 w257]
        frame False {
          n164 = call <vilib>:"WPI_MotorControlSetOutput.vi"("Output"=0.0, "MotorControlDevRef"=w255) -> ()  [unwired: 7 in, 3 out]
        }
        frame True {
          n165 = call <vilib>:"WPI_MotorControlSetOutput.vi"("Output"=-1.0, "MotorControlDevRef"=w257) -> ()  [unwired: 7 in, 3 out]
        }
      }
    }
    frame True {
      n166 = case shown="True" w259 {
        tunnel: w258 -> [w261 w263]
        frame False {
          n167 = call <vilib>:"WPI_MotorControlSetOutput.vi"("Output"=1.0, "MotorControlDevRef"=w261) -> ()  [unwired: 7 in, 3 out]
        }
        frame True {
          n168 = call <vilib>:"WPI_MotorControlSetOutput.vi"("Output"=0.0, "MotorControlDevRef"=w263) -> ()  [unwired: 7 in, 3 out]
        }
      }
    }
  }
  n169 = call <vilib>:"WPI_DigitalInputGetValue.vi"("DigitalInputDevRef"=w21) -> ("Value"=w22:bool)  [unwired: 8 in, 2 out]
  n170 = Negate(x=w60) -> (-x=w59:dbl)
  n171 = call <vilib>:"WPI_DigitalInputRefNum Registry Get.vi"("refnum name"="Bottom Limit Switch") -> ("DigitalInputDevRef"=w25:T27)  [unwired: 9 in, 1 out]
  n172 = call <vilib>:"WPI_DigitalInputRefNum Registry Get.vi"("refnum name"="Top Limit Switch") -> ("DigitalInputDevRef"=w18:T27)  [unwired: 9 in, 1 out]
  n173 = call <vilib>:"WPI_DigitalInputGetValue.vi"("DigitalInputDevRef"=w25) -> ("Value"=w13:bool)  [unwired: 8 in, 2 out]
  n174 = call <vilib>:"WPI_DigitalInputGetValue.vi"("DigitalInputDevRef"=w18) -> ("Value"=w8:bool)  [unwired: 8 in, 2 out]
  n175 = Negate(x=w90) -> (-x=w89:dbl)
  n176 = Negate(x=w88) -> (-x=w87:dbl)
  n177 = call <vilib>:"SD Write Numeric Array.vi"("Numeric Array"=w119, "Name"="Joystick 1/Axes") -> ()  [unwired: 8 in, 2 out]
  n178 = call <vilib>:"WPI_RobotDriveRefNum Registry Get.vi"("refnum name"="Left and Right Motors") -> ("RobotDriveDevRef"=w127:T35)  [unwired: 1 in, 9 out]
  n179 = Not(x=w22) -> (.not. x?=w12:bool)
  n180 = Multiply(x=w59, y=0.4) -> (x*y=w9:dbl)
  n181 = call <vilib>:"WPI_EncoderRefNum Registry Get.vi"("refnum name"="Left Drive Encoder") -> ("EncoderDevRef"=w5:T15)  [unwired: 9 in, 1 out]
  n182 = call <vilib>:"WPI_EncoderRefNum Registry Get.vi"("refnum name"="Right Drive Encoder") -> ("error out"=w7:errorcluster, "EncoderDevRef"=w6:T15)  [unwired: 9 in]
  n183 = call <vilib>:"WPI_RobotDriveArcadeDrive_Standard(NoSaturation).vi"("Y axis value"=w87, "X axis value"=w89, "RobotDriveDevRef"=w127) -> ("Motor Values"=w116:dbl[])  [unwired: 1 in, 7 out]
  n184 = call <vilib>:"WPI_EncoderGet.vi"("error in (no error)"=w7, "EncoderDevRef"=w6) -> ("Distance"=→"Waveform Chart 3":dbl)  [unwired: 4 in, 5 out]
  n185 = Less?(x=w9, y=-0.01) -> (x < y?=w24:bool)
  n186 = And(x=w13, y=w12) -> (x .and. y?=w11:bool)
  n187 = And(x=w8, y=w12) -> (x .and. y?=w16:bool)
  n188 = call <vilib>:"SD Write Numeric Array.vi"("Numeric Array"=w116, "Name"="Robot Drive Motors") -> ()  [unwired: 8 in, 2 out]
  n189 = call <vilib>:"WPI_EncoderGet.vi"("EncoderDevRef"=w5) -> ("Distance"=→"Waveform Chart 2":dbl)  [unwired: 5 in, 5 out]
  n190 = Greater?(x=w9, y=0.01) -> (0:w17:bool)
  n191 = And(x=w11, y=w24) -> (x .and. y?=w14:bool)
  n192 = And(x=w17, y=w16) -> (x .and. y?=w15:bool)
  n193 = call <vilib>:"SD Write Boolean Array.vi"("Boolean Array"=w122, "Name"="Joystick 1/Buttons") -> ()  [unwired: 8 in, 2 out]
  n194 = Or(x=w14, y=w15) -> (x .or. y?=w10:bool)
  n195 = case shown="False" w10 {
    tunnel: w9 -> [_ w267]
    frame False {
      n196 = call <vilib>:"WPI_MotorControlRefNum Registry Get.vi"("refnum name"="Fisher Price") -> ("MotorControlDevRef"=w265:T8)  [unwired: 9 in, 1 out]
      n197 = call <vilib>:"WPI_MotorControlSetOutput.vi"("Output"=0.0, "MotorControlDevRef"=w265) -> ()  [unwired: 7 in, 3 out]
    }
    frame True {
      n198 = call <vilib>:"WPI_MotorControlRefNum Registry Get.vi"("refnum name"="Fisher Price") -> ("MotorControlDevRef"=w269:T8)  [unwired: 9 in, 1 out]
      n199 = call <vilib>:"WPI_MotorControlSetOutput.vi"("Output"=w267, "MotorControlDevRef"=w269) -> ()  [unwired: 7 in, 3 out]
    }
  }
